vi "niRFUtil RFHS Channelizer FrequencyShiftInitialize CSG.vi"(0 "fc":dbl) -> (4 "Float Cache":csg[](array[numeric]), 6 "Double Cache":cdb[](array[numeric]))   [LabVIEW 2015, in "niRFUtil.lvlib"]
uses:
  niRFUtil.lvlib
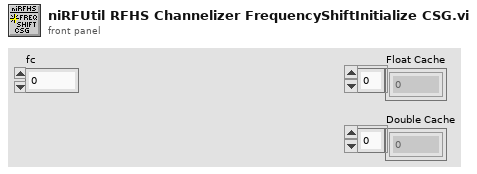
[diagram p1: front panel]
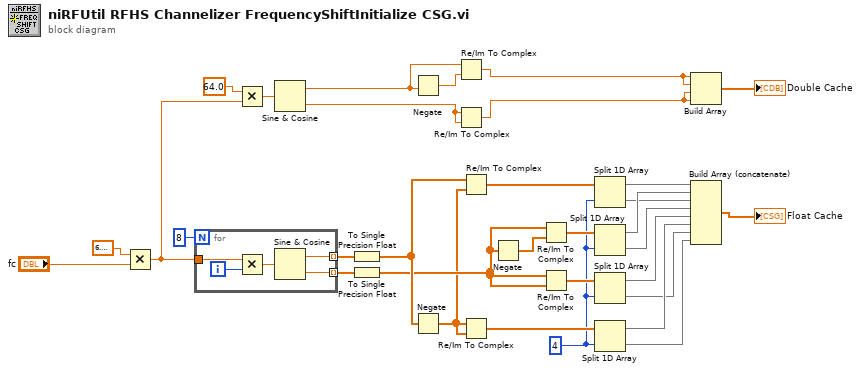
[diagram p0: block diagram]
diagram:
  w15 = 4 ("index")
  n1 = Multiply(x=6.283185307179586, y="fc") -> (x*y=w27:dbl)
  n2 = for {
    N: 8 -> [_]
    tunnel: w27 -> [w37]
    tunnel: [w34] -> w25 mode=indexing
    tunnel: [w33] -> w24 mode=indexing
    i -> [w36]
    n3 = Multiply(x=w37, y=w36) -> (x*y=w35:dbl)
    n4 = Sine & Cosine(0:w35) -> (1:w34:dbl, 2:w33:dbl)
  }
  n5 = Multiply(x=64.0 ("value"), y=w27) -> (x*y=w29:dbl)
  n6 = Sine & Cosine(0:w29) -> (1:w4:dbl, 2:w6:dbl)
  n7 = To Single Precision Float(number=w25) -> (single precision float=w23:sgl[])
  n8 = To Single Precision Float(number=w24) -> (single precision float=w21:sgl[])
  n9 = Negate(x=w4) -> (-x=w5:dbl)
  n10 = Negate(x=w23) -> (-x=w20:sgl[])
  n11 = Re/Im To Complex(1:w5, 2:w4) -> (0:w3:cdb)
  n12 = Re/Im To Complex(1:w6, 2:w6) -> (0:w1:cdb)
  n13 = Re/Im To Complex(1:w20, 2:w23) -> (0:w19:csg[])
  n14 = Re/Im To Complex(1:w20, 2:w20) -> (0:w16:csg[])
  n15 = Negate(x=w21) -> (-x=w22:sgl[])
  n16 = Re/Im To Complex(1:w22, 2:w21) -> (0:w18:csg[])
  n17 = Re/Im To Complex(1:w21, 2:w21) -> (0:w17:csg[])
  n18 = Split 1D Array(array=w19, index=w15) -> (first subarray=w14:csg[], second subarray=w12:csg[])
  n19 = Split 1D Array(array=w18, index=w15) -> (first subarray=w13:csg[], second subarray=w11:csg[])
  n20 = Split 1D Array(array=w17, index=w15) -> (first subarray=w10:csg[], second subarray=w8:csg[])
  n21 = Split 1D Array(array=w16, index=w15) -> (first subarray=w9:csg[], second subarray=w7:csg[])
  n22 = Build Array(w3, w3, w1, w1) -> (→"Double Cache":cdb[])
  n23 = Build Array (concatenate)(w14, w13, w12, w11, w10, w9, w8, w7) -> (→"Float Cache":csg[])
